vi "Cleanup Instrument Engine.vi"(8 "error in (no error)":errorcluster, 11 "State Variables":T1) -> ()   [LabVIEW 2018, in "Instrument Addon Engine.lvlib"]
uses:
  Instrument Addon Engine.lvlib
  <vilib>/NI/NI VeriStand Addon Network Comm/Engine/VeriStand Comm.lvclass
  Types/Engine State Variables.ctl
  <vilib>/NI/NIVS Inline Async API/_VS Inline Async API/Process/Process.lvclass
  <vilib>/NI/NIVS Inline Async API/_Data Access Engine/Access Type Classes/ReadWrite/ReadWrite.lvclass
  <vilib>/NI/NIVS Inline Async API/_Data Access Engine/Access Type Classes/Write/Write.lvclass
  <vilib>/NI/NIVS Inline Async API/_Data Access Engine/Data Access Engine/Types/Write.DVR.ctl
  <vilib>/NI/NIVS Inline Async API/_Data Access Engine/Data Access Engine/Data Access Engine.lvclass
  <vilib>/NI/NIVS Inline Async API/_Data Access Engine/Access Type Classes/Read/Read.lvclass
  <vilib>/NI/NIVS Inline Async API/_Data Access Engine/Data Access Engine/Types/Read.DVR.ctl
  <vilib>/NI/NIVS Inline Async API/_Data Access Engine/Data Access Engine/Types/ReadWrite.DVR.ctl
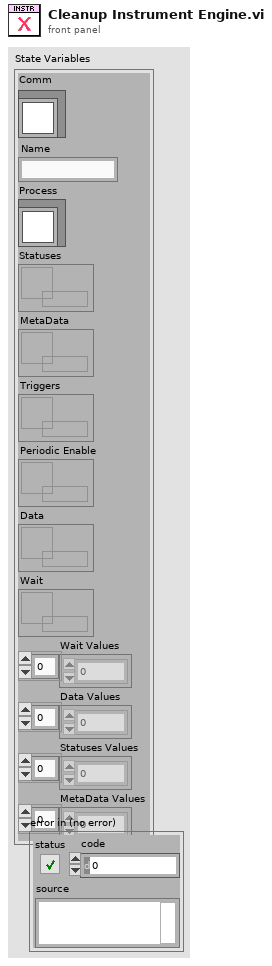
[diagram p1: front panel]
types:
  T1 = typedef "Instrument Addon Engine.lvlib/Engine State Variables.ctl" = cluster{"Comm":refnum<class "VeriStand Comm.lvclass">, "Name":string, "Process":refnum<class "Process.lvclass">, "Statuses":T2, "MetaData":T3, "Triggers":T4, "Periodic Enable":T3, "Data":T2, "Wait":T3, "Wait Values":dbl[], "Data Values":dbl[], "Statuses Values":dbl[], "MetaData Values":dbl[]}
  T2 = typedef "Data Access Engine.lvlib/Data Access Engine.lvclass/Write.DVR.ctl" = refnum<data-value>
  T3 = typedef "Data Access Engine.lvlib/Data Access Engine.lvclass/Read.DVR.ctl" = refnum<data-value>
  T4 = typedef "Data Access Engine.lvlib/Data Access Engine.lvclass/ReadWrite.DVR.ctl" = refnum<data-value>
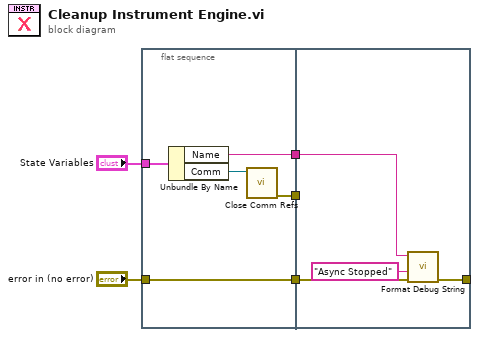
[diagram p0: block diagram]
diagram:
  n1 = flat-sequence {
    tunnel: "error in (no error)" -> [w8]
    tunnel: "State Variables" -> [w10]
    tunnel: [w9] -> w5
    tunnel: [w8] -> w2
    tunnel: [w6] -> w1
    tunnel: w5 -> [_]
    tunnel: w2 -> [w12]
    tunnel: w1 -> [w14]
    tunnel: [w11] -> _
    frame #0 {
      n2 = Unbundle By Name(w10) -> ("Name"=w6:string, "Comm"=w7:refnum<class "VeriStand Comm.lvclass">)
      n3 = call <vilib>:"Close Comm Refs.vi"("Comm.lvclass"=w7) -> ("error out"=w9:errorcluster)  [unwired: 10 in]
    }
    frame #1 {
      n4 = call "Format Debug String.vi"("error in (no error)"=w12, "State"="Async Stopped", "Name"=w14) -> ("error out"=w11:errorcluster)  [unwired: 8 in]
    }
  }
